vi "Initialise DVR's.vi"(8 "error in (no error)":errorcluster) -> (0 "error out":errorcluster, 3 "Type":T1)   [LabVIEW 2021, in "Fault-Injection Bus.lvclass"]
uses:
  Fault-Injection Bus.lvclass
  DVR Type.ctl
  Value Type/Boolean/Support/DVR Type.ctl
  Value Type/Boolean/Support/Value Type.ctl
  Value Type/DBL/Support/DVR Type.ctl
  Value Type/DBL/Support/Value Type.ctl
  Fault-Injection Bus.lvclass/Fault-Injection Bus.ctl
  <vilib>/TSA/Abstract Data Classes/Abs_Types/Type/Abs_Type.lvclass
  Value Type/Boolean/Fault-Injection_Boolean.lvclass
  <vilib>/TSA/Abstract Data Classes/Abs_Types/Boolean/Abs_Boolean.lvclass
  <vilib>/TSA/Abstract Data Classes/Abs_Types/Double Float/Abs_Double Float.lvclass
  Value Type/DBL/Fault-Injection_DBL.lvclass
  <vilib>/TSA/Abstract Data Classes/Abs_Types/Single Float/Abs_Single Float.lvclass
  Value Type/SGL/Support/Value Type.ctl
  Value Type/SGL/Fault-Injection_SGL.lvclass
  Value Type/SGL/Support/DVR Type.ctl
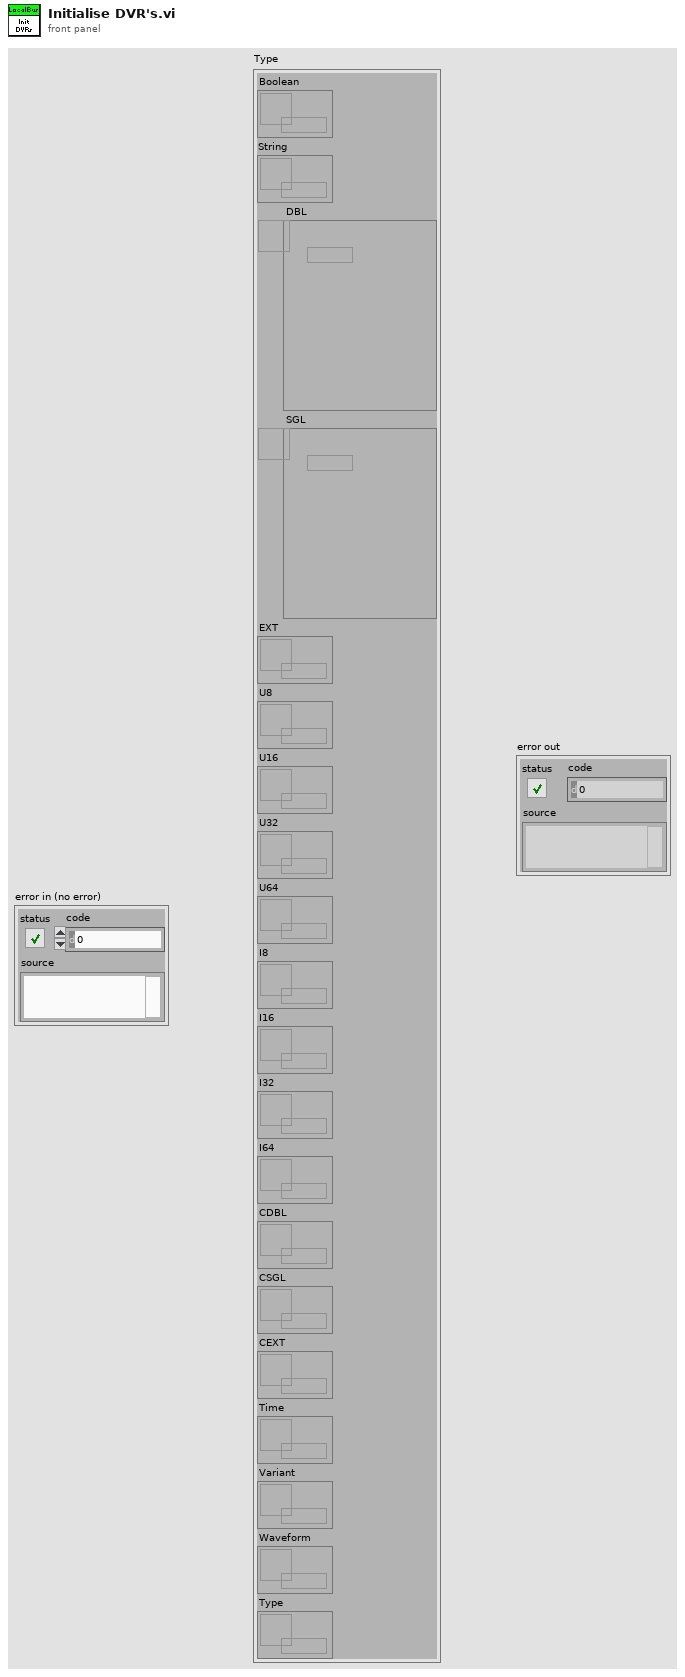
[diagram p1: front panel]
types:
  T1 = typedef "Fault-Injection Bus.lvclass/DVR Type.ctl" = cluster{"Boolean":refnum<data-value>, "String":refnum<data-value>, "DBL":refnum<data-value>, "SGL":refnum<data-value>, "EXT":refnum<data-value>, "U8":refnum<data-value>, "U16":refnum<data-value>, "U32":refnum<data-value>, "U64":refnum<data-value>, "I8":refnum<data-value>, "I16":refnum<data-value>, "I32":refnum<data-value>, "I64":refnum<data-value>, "CDBL":refnum<data-value>, "CSGL":refnum<data-value>, "CEXT":refnum<data-value>, "Time":refnum<data-value>, "Variant":refnum<data-value>, "Waveform":refnum<data-value>, "Type":refnum<data-value>}
  T2 = typedef "Fault-Injection_SGL.lvclass/DVR Type.ctl" = cluster{"Enable":bool, "Injected Value":T3, "Value":refnum<class "Abs_Single Float.lvclass">}
  T3 = typedef "Fault-Injection_SGL.lvclass/Value Type.ctl" = sgl
  T4 = typedef "Fault-Injection_DBL.lvclass/DVR Type.ctl" = cluster{"Enable":bool, "Injected Value":T5, "Value":refnum<class "Abs_Double Float.lvclass">}
  T5 = typedef "Fault-Injection_DBL.lvclass/Value Type.ctl" = dbl
  T6 = typedef "Fault-Injection_Boolean.lvclass/DVR Type.ctl" = cluster{"Enable":bool, "Injected Value":T7, "Value":refnum<class "Abs_Boolean.lvclass">}
  T7 = typedef "Fault-Injection_Boolean.lvclass/Value Type.ctl" = bool
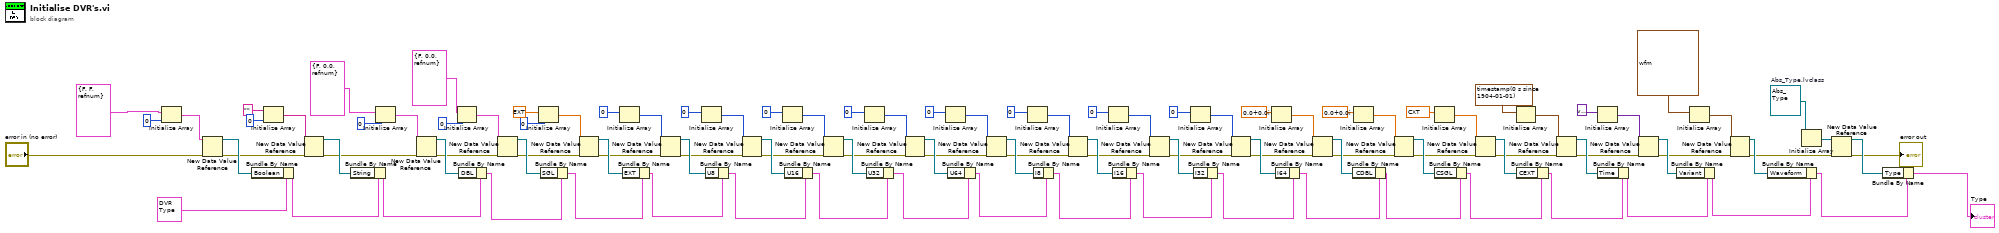
[diagram p0: block diagram]
diagram:
  w13 = refnum<class "Abs_Type.lvclass"> refnum  # Abs_Type.lvclass
  n1 = Initialize Array(T6 {"Enable"=FALSE, "Injected Value"=FALSE, "Value"=refnum} ("Cluster"), 0 ("dimension size")) -> (w107:T6[])
  n2 = New Data Value Reference(data value=w107, error in="error in (no error)") -> (data value reference=w105:refnum<data-value>, error out=w102:errorcluster)
  n3 = Bundle By Name(cluster=T1 {"Boolean"=refnum, "String"=refnum, "DBL"=refnum, "SGL"=refnum, "EXT"=refnum, "U8"=refnum, "U16"=refnum, "U32"=refnum, "U64"=refnum, "I8"=refnum, "I16"=refnum, "I32"=refnum, "I64"=refnum, "CDBL"=refnum, "CSGL"=refnum, "CEXT"=refnum, "Time"=refnum, "Variant"=refnum, "Waveform"=refnum, "Type"=refnum} ("Type"), "Boolean"=w105) -> (w104:T1)
  n4 = Initialize Array("", 0 ("dimension size")) -> (w103:string[])
  n5 = New Data Value Reference(data value=w103, error in=w102) -> (data value reference=w100:refnum<data-value>, error out=w97:errorcluster)
  n6 = Bundle By Name(cluster=w104, "String"=w100) -> (w96:T1)
  n7 = Initialize Array(T4 {"Enable"=FALSE, "Injected Value"=0.0, "Value"=refnum} ("Cluster"), 0 ("dimension size")) -> (w98:T4[])
  n8 = New Data Value Reference(data value=w98, error in=w97) -> (data value reference=w99:refnum<data-value>, error out=w32:errorcluster)
  n9 = Initialize Array(T2 {"Enable"=FALSE, "Injected Value"=0.0, "Value"=refnum} ("Cluster"), 0 ("dimension size")) -> (w95:T2[])
  n10 = Bundle By Name(cluster=w96, "DBL"=w99) -> (w75:T1)
  n11 = New Data Value Reference(data value=w95, error in=w32) -> (data value reference=w94:refnum<data-value>, error out=w31:errorcluster)
  n12 = Initialize Array(ext 0.0, 0 ("dimension size")) -> (w92:ext[])
  n13 = Bundle By Name(cluster=w75, "SGL"=w94) -> (w74:T1)
  n14 = New Data Value Reference(data value=w92, error in=w31) -> (data value reference=w93:refnum<data-value>, error out=w30:errorcluster)
  n15 = Initialize Array(u8 0) -> (w89:u8[])  [unwired: 1 in]
  n16 = Bundle By Name(cluster=w74, "EXT"=w93) -> (w73:T1)
  n17 = New Data Value Reference(data value=w89, error in=w30) -> (data value reference=w88:refnum<data-value>, error out=w29:errorcluster)
  n18 = Initialize Array(u16 0) -> (w77:u16[])  [unwired: 1 in]
  n19 = Bundle By Name(cluster=w73, "U8"=w88) -> (w72:T1)
  n20 = New Data Value Reference(data value=w77, error in=w29) -> (data value reference=w76:refnum<data-value>, error out=w28:errorcluster)
  n21 = Initialize Array(u32 0) -> (w80:u32[])  [unwired: 1 in]
  n22 = Bundle By Name(cluster=w72, "U16"=w76) -> (w71:T1)
  n23 = New Data Value Reference(data value=w80, error in=w28) -> (data value reference=w81:refnum<data-value>, error out=w27:errorcluster)
  n24 = Initialize Array(u64 0) -> (w83:u64[])  [unwired: 1 in]
  n25 = Bundle By Name(cluster=w71, "U32"=w81) -> (w70:T1)
  n26 = New Data Value Reference(data value=w83, error in=w27) -> (data value reference=w82:refnum<data-value>, error out=w26:errorcluster)
  n27 = Initialize Array(i8 0) -> (w86:i8[])  [unwired: 1 in]
  n28 = Bundle By Name(cluster=w70, "U64"=w82) -> (w46:T1)
  n29 = New Data Value Reference(data value=w86, error in=w26) -> (data value reference=w87:refnum<data-value>, error out=w25:errorcluster)
  n30 = Initialize Array(i16 0) -> (w49:i16[])  [unwired: 1 in]
  n31 = Bundle By Name(cluster=w46, "I8"=w87) -> (w45:T1)
  n32 = New Data Value Reference(data value=w49, error in=w25) -> (data value reference=w48:refnum<data-value>, error out=w24:errorcluster)
  n33 = Initialize Array(0) -> (w51:i32[])  [unwired: 1 in]
  n34 = Bundle By Name(cluster=w45, "I16"=w48) -> (w44:T1)
  n35 = New Data Value Reference(data value=w51, error in=w24) -> (data value reference=w52:refnum<data-value>, error out=w23:errorcluster)
  n36 = Initialize Array(i64 0) -> (w54:i64[])  [unwired: 1 in]
  n37 = Bundle By Name(cluster=w44, "I32"=w52) -> (w43:T1)
  n38 = New Data Value Reference(data value=w54, error in=w23) -> (data value reference=w53:refnum<data-value>, error out=w22:errorcluster)
  n39 = Initialize Array(cdb 0.0+0.0i) -> (w57:cdb[])  [unwired: 1 in]
  n40 = Bundle By Name(cluster=w43, "I64"=w53) -> (w42:T1)
  n41 = New Data Value Reference(data value=w57, error in=w22) -> (data value reference=w58:refnum<data-value>, error out=w21:errorcluster)
  n42 = Bundle By Name(cluster=w42, "CDBL"=w58) -> (w41:T1)
  n43 = Initialize Array(csg 0.0+0.0i) -> (w68:csg[])  [unwired: 1 in]
  n44 = New Data Value Reference(data value=w68, error in=w21) -> (data value reference=w69:refnum<data-value>, error out=w20:errorcluster)
  n45 = Bundle By Name(cluster=w41, "CSGL"=w69) -> (w40:T1)
  n46 = Initialize Array(cxt 0.0+0.0i) -> (w65:cxt[])  [unwired: 1 in]
  n47 = New Data Value Reference(data value=w65, error in=w20) -> (data value reference=w64:refnum<data-value>, error out=w19:errorcluster)
  n48 = Initialize Array(timestamp(0 s since 1904-01-01)) -> (w62:timestamp[])  [unwired: 1 in]
  n49 = Bundle By Name(cluster=w40, "CEXT"=w64) -> (w39:T1)
  n50 = New Data Value Reference(data value=w62, error in=w19) -> (data value reference=w63:refnum<data-value>, error out=w18:errorcluster)
  n51 = Initialize Array(variant) -> (w60:variant[])  [unwired: 1 in]
  n52 = Bundle By Name(cluster=w39, "Time"=w63) -> (w38:T1)
  n53 = New Data Value Reference(data value=w60, error in=w18) -> (data value reference=w59:refnum<data-value>, error out=w17:errorcluster)
  n54 = Bundle By Name(cluster=w38, "Variant"=w59) -> (w36:T1)
  n55 = Initialize Array(waveform(dbl) {"t0"=timestamp(0 s since 1904-01-01), "dt"=1.0, "Y"=[]}) -> (w37:waveform(dbl)[])  [unwired: 1 in]
  n56 = New Data Value Reference(data value=w37, error in=w17) -> (data value reference=w35:refnum<data-value>, error out=w12:errorcluster)
  n57 = Bundle By Name(cluster=w36, "Waveform"=w35) -> (w16:T1)
  n58 = Initialize Array(w13) -> (w14:refnum<class "Abs_Type.lvclass">[])  [unwired: 1 in]
  n59 = New Data Value Reference(data value=w14, error in=w12) -> (data value reference=w15:refnum<data-value>, error out=→"error out":errorcluster)
  n60 = Bundle By Name(cluster=w16, "Type"=w15) -> (→"Type":T1)
